vi "RT Main_FPGA Interface.vi"() -> ()   [LabVIEW 2018]
uses:
  TypeDefs/Simple cluster.ctl
  <vilib>/FPGAPlugInAG/cRIO-9039 (Sync)/niLvFpga_Open_cRIO-9039 (Sync).vi
  <vilib>/rvi/interface/common/dynamic/niFpgaDynamicAddResources.vi
  <vilib>/Utility/error.llb/Error Cluster From Error Code.vi
  <vilib>/rvi/errors/niLvFpgaAdjustHostInterfaceError.vi
  <vilib>/FPGAPlugInAG/Dynamic/niLvFpga_Close_Dynamic.vi
  <vilib>/rvi/interface/nirviOpenFPGA/nirviOpenFPGA.xnode
  cRIO FPGA/FPGA Bitfiles/Scalar FPGA Personality.lvbitx
  <vilib>/rvi/interface/nirviReadWriteControl/nirviReadWriteControl.xnode
  <vilib>/rvi/interface/nirviCloseFPGA/nirviCloseFPGA.xnode
  NiFpgaLv.dll
  <vilib>/rvi/interface/Simulation/niFpgaSimulationCallBeginRW.vi
panel:
  out "error out":errorcluster
  out "Average seconds per read":dbl format="%#_6f"
  out "Cluster out":T1
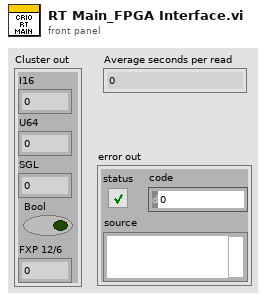
[diagram p1: front panel]
types:
  T1 = typedef "Simple cluster.ctl" = cluster{"I16":i16, "U64":u64, "SGL":sgl, "Bool":bool, "FXP 12/6":fxp<+/-,12,6>}
  T2 = cluster{"I16":i16, "U64":u64, "SGL":sgl, "Bool":bool, "FXP 12/6":fxp<+/-,12,6>}
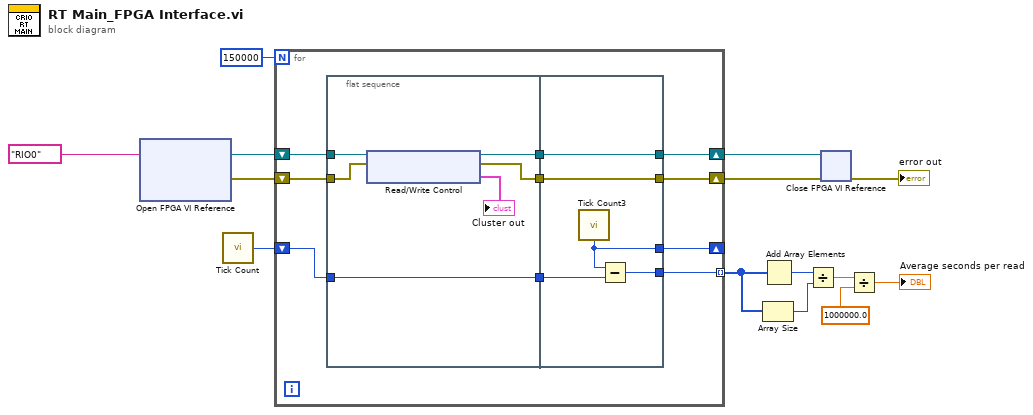
[diagram p0: block diagram]
diagram:
  n1 = xnode "Open FPGA VI Reference"("resource name"=tag "RIO0") -> ("FPGA VI Reference Out"=w12:refnum<k20>, "error out"=w13:errorcluster)  [unwired: 1 in]
  n2 = call "Tick Count"() -> ("Tick Count(uSec)"=w1:u32)
  n3 = for {
    N: 150000 -> [_]
    shift-right: [w15] -> w11
    shift-left: w13 -> [w24]
    shift-right: [w21] -> _
    shift-left: w1 -> [w23]
    tunnel: [w20] -> w5 mode=indexing
    shift-right: [w17] -> w10
    shift-left: w12 -> [w19]
    n4 = flat-sequence {
      tunnel: w24 -> [w28]
      tunnel: w23 -> [w30]
      tunnel: [w30] -> w22
      tunnel: w19 -> [w29]
      tunnel: [w27] -> w18
      tunnel: [w26] -> w16
      tunnel: w22 -> [w35]
      tunnel: [w34] -> w21
      tunnel: [w33] -> w20
      tunnel: [w32] -> w17
      tunnel: w18 -> [w32]
      tunnel: w16 -> [w31]
      tunnel: [w31] -> w15
      frame #0 {
        n5 = xnode "Read/Write Control"("FPGA VI Reference In"=w29, "error in"=w28) -> ("FPGA VI Reference Out"=w27:refnum<k20>, "error out"=w26:errorcluster, "Simple cluster out"=→"Cluster out":T2)
      }
      frame #1 {
        n6 = call "Tick Count3"() -> ("Tick Count(uSec)"=w34:u32)
        n7 = Subtract(x=w34, y=w35) -> (x-y=w33:u32)
      }
    }
  }
  n8 = Array Size(array=w5) -> (size(s)=w7:i32)
  n9 = Add Array Elements(numeric array=w5) -> (sum=w6:u32)
  n10 = Divide(x=w6, y=w7) -> (x/y=w8:dbl)
  n11 = xnode "Close FPGA VI Reference"("FPGA VI Reference In"=w10, "error in"=w11) -> ("error out"=→"error out":errorcluster)
  n12 = Divide(x=w8, y=1000000.0) -> (x/y=→"Average seconds per read":dbl)
